vi "Configure Modulation.vi"   [LabVIEW 2012, in "Agilent PSG MXG Series.lvlib"]
doc: "Configures amplitude modulation, frequency modulation, phase modulation, pulse modulation, I/Q modulation, custom(advanced) modulation, digital modulation and wideband I/Q modulation, LF Output modulation."
uses:
  <instrlib>/Agilent PSG MXG Series/Agilent PSG MXG Series.lvlib
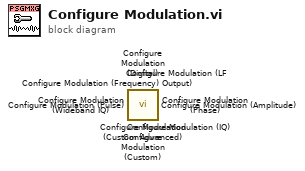
[diagram p0: block diagram]
diagram:
  n1 = call <instrlib>:"Configure Modulation (Custom Advanced).vi"() -> ()  [unwired: 14 in, 2 out]
  n2 = call <instrlib>:"Configure Modulation (LF Output).vi"() -> ()  [unwired: 14 in, 2 out]
  n3 = call <instrlib>:"Configure Modulation (Wideband IQ).vi"() -> ()  [unwired: 14 in, 2 out]
  n4 = call <instrlib>:"Configure Modulation (Phase).vi"() -> ()  [unwired: 14 in, 2 out]
  n5 = call <instrlib>:"Configure Modulation (Frequency).vi"() -> ()  [unwired: 14 in, 2 out]
  n6 = call <instrlib>:"Configure Modulation (Digital).vi"() -> ()  [unwired: 14 in, 2 out]
  n7 = call <instrlib>:"Configure Modulation (Custom).vi"() -> ()  [unwired: 14 in, 2 out]
  n8 = call <instrlib>:"Configure Modulation (IQ).vi"() -> ()  [unwired: 14 in, 2 out]
  n9 = call <instrlib>:"Configure Modulation (Pulse).vi"() -> ()  [unwired: 14 in, 2 out]
  n10 = call <instrlib>:"Configure Modulation (Amplitude).vi"() -> ()  [unwired: 14 in, 2 out]
